vi "Enable_Current_Protection.vi"(8 "error in (no error)":errorcluster caption="entrée d'erreur (pas d'erreur)", 11 "Class Power_Supply Rigol DP800 en entrée":refnum<class "Class Power_Supply Rigol DP800.lvclass">) -> (0 "error out":errorcluster caption="sortie d'erreur", 3 "Class Power_Supply Rigol DP800 en sortie":refnum<class "Class Power_Supply Rigol DP800.lvclass">)   [LabVIEW 2020, in "Library Instrument & Equipement.lvlib" / "Library Power_Supply.lvlib" / "Class Power_Supply Rigol DP800.lvclass"]
uses:
  Class Power_Supply Rigol DP800.lvclass
  C:/Users/ngarcin/OneDrive - Altyor/Standard TB/Class/Power_Supply/Power_Supply (Default)/Power_Supply (Default).lvclass
  Class Power_Supply Rigol DP800.lvclass/Class Power_Supply Rigol DP800.ctl
  RIGOL DP800 Series/RIGOL DP800 Series.lvlib
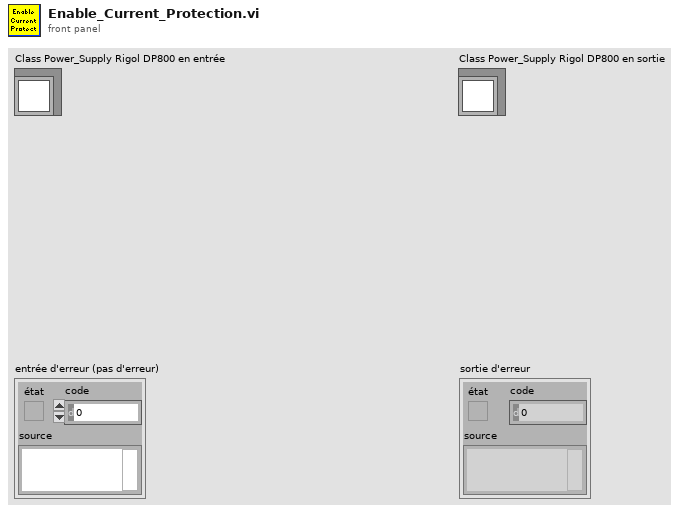
[diagram p1: front panel]
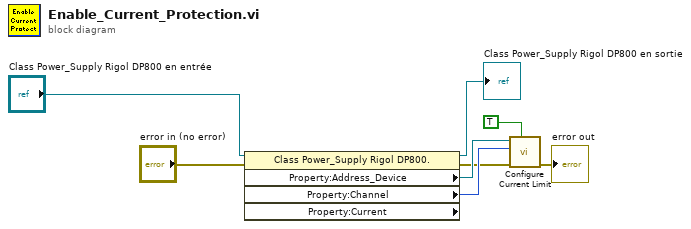
[diagram p0: block diagram]
diagram:
  n1 = property class="Class Power_Supply Rigol DP800." props=["Property:Address_Device", "Property:Channel", "Property:Current"](reference="Class Power_Supply Rigol DP800 en entrée", error in="error in (no error)") -> (reference out=→"Class Power_Supply Rigol DP800 en sortie":refnum<class "Class Power_Supply Rigol DP800.lvclass">, error out=w2:errorcluster, "Property:Address_Device"=w8:refnum<visa-resource-name>, "Property:Channel"=w7:i32)  [unwired: 1 out]
  n2 = call "Configure Current Limit.vi"("Enable OCP (T: Enable)"=TRUE, "error in (no error)"=w2, "Channel (0: 30V Channel)"=w7, "VISA resource name"=w8) -> ("error out"=→"error out":errorcluster)  [unwired: 6 in, 1 out]
